vi "Open Loop Shooter Control.vi"() -> (2 "Open Loop PWM":dbl)   [LabVIEW 2011]
uses:
  System Set Points and States.vi
panel:
  # "0.5 from the key to high goal"
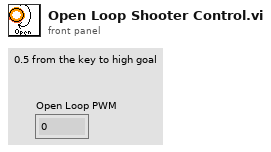
[diagram p1: front panel]
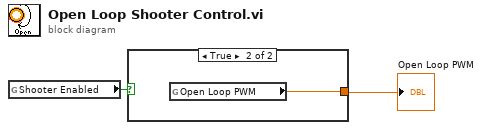
[diagram p0: block diagram]
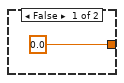
[diagram p2: hidden frame]
diagram:
  n1 = global read "System Set Points and States.vi" "Shooter Enabled"() -> (w2:bool)
  n2 = case shown="True" w2 {
    tunnel: [0.0 w4] -> w1
    frame False {
    }
    frame True {
      n3 = global read "System Set Points and States.vi" "Open Loop PWM"() -> (w4:dbl)
    }
  }
  "Open Loop PWM" <- w1
